vi "MB Ethernet Master Query Write Multiple Registers (poly).vi"(0 "TCP Connection Refnum in":refnum<k5>, 1 "Starting Address":u16, 2 "Registers":u16[](array[numeric]), 4 "Timeout":u32=10000, 5 "error in":errorcluster, 6 "MBAP Header":cluster{"Transaction ID":u16, "Unit ID":u8}) -> (14 "TCP Connection Refnum (dup)":refnum<k5>, 16 "Exception Code":u8 format="%.0x", 19 "error out":errorcluster)   [LabVIEW 2011]
doc: "The master uses this VI to write multiple registers to the slave. This corresponds to a public function code of 16 in the MODBUS protocol."
uses:
  MB Modbus Command.ctl
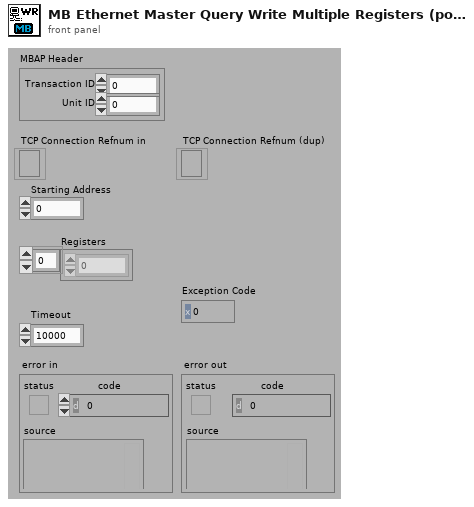
[diagram p1: front panel]
types:
  T1 = typedef "MB Modbus Command.ctl" = cluster{"Function Code":u8, "Starting Address":u16, "Quantity":u16, "Data":u16[], "Discrete":bool[]}
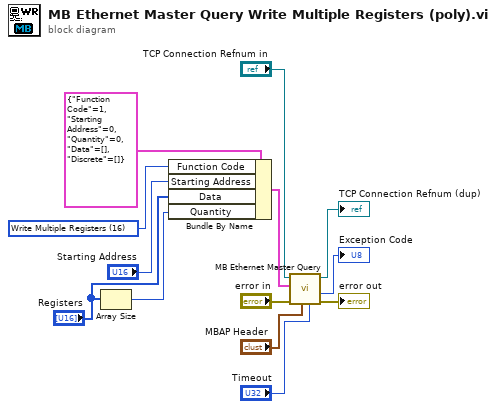
[diagram p0: block diagram]
diagram:
  w11 = u8 16 items=["Read Coils"=1, "Read Discrete Inputs"=2, "Read Holding Registers"=3, "Read Input Registers"=4, "Write Single Coil"=5, "Write Single Register"=6, "Read Exception Status"=7, "Write Multiple Coils"=15, "Write Multiple Registers"=16] ("Function Code")
  n1 = Array Size(array="Registers") -> (size(s)=w1:i32)
  n2 = Bundle By Name(cluster=T1 {"Function Code"=1, "Starting Address"=0, "Quantity"=0, "Data"=[], "Discrete"=[]} ("Modbus Command"), "Function Code"=w11, "Starting Address"="Starting Address", "Data"="Registers", "Quantity"=w1) -> (w12:T1)
  n3 = call "MB Ethernet Master Query.vi"("Timeout"="Timeout", "MBAP Header"="MBAP Header", "error in (no error)"="error in", "Modbus Command"=w12, "TCP Connection Refnum in"="TCP Connection Refnum in") -> ("error out"=→"error out":errorcluster, "Exception Code"=→"Exception Code":u8, "TCP Connection Refnum (dup)"=→"TCP Connection Refnum (dup)":refnum<k5>)  [unwired: 2 in, 2 out]
